vi "getAllsubset.vi"(8 "error in (no error)":errorcluster, 10 "getAll":T1, 11 "instrument.OptiCool in":refnum<class "instrument.OptiCool.lvclass">) -> (0 "error out":errorcluster, 2 "output cluster":variant, 3 "instrument.OptiCool out":refnum<class "instrument.OptiCool.lvclass">)   [LabVIEW 2019, in "instrument.OptiCool.lvclass"]
uses:
  instrument.OptiCool.lvclass
  instrument.PPMS/Typedefs/PPMS.getAll--cluster.ctl
  instrument.PPMS/instrument.PPMS.lvclass
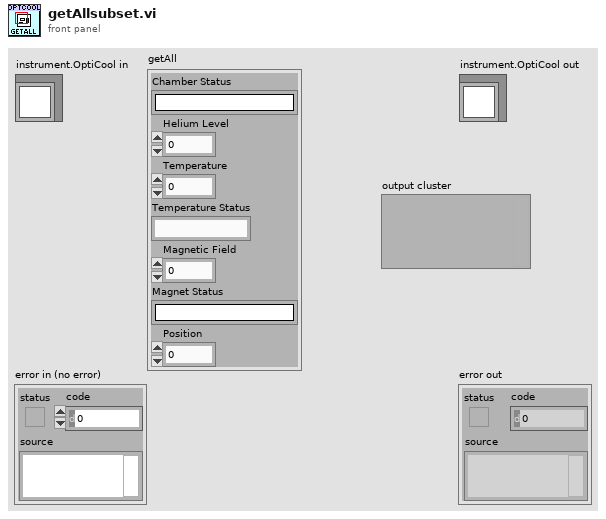
[diagram p1: front panel]
types:
  T1 = typedef "instrument.PPMS.lvclass/PPMS.getAll--cluster.ctl" = cluster{"Chamber Status":string, "Helium Level":dbl, "Temperature":dbl, "Temperature Status":string, "Magnetic Field":dbl, "Magnet Status":string, "Position":dbl}
  T2 = cluster{"Chamber Status":string, "Temperature":dbl, "Temperature Status":string, "Magnetic Field":dbl, "Magnet Status":string}
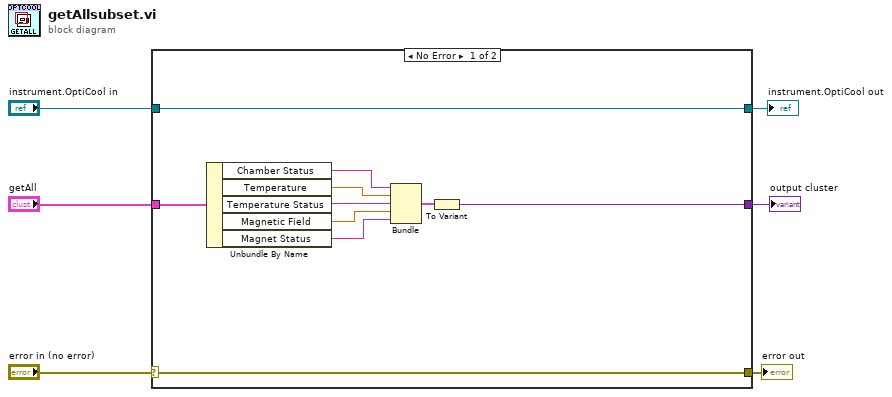
[diagram p0: block diagram]
diagram:
  n1 = case shown="No Error" "error in (no error)" {
    selector: "error in (no error)" -> [w15 w18]
    tunnel: [w15 w18] -> w1
    tunnel: [w16 w17] -> w2
    tunnel: "instrument.OptiCool in" -> [w16 w17]
    tunnel: "getAll" -> [w8 _]
    tunnel: [w14 _] -> w3
    frame No Error {
      n2 = Unbundle By Name(w8) -> ("Chamber Status"=w11:string, "Temperature"=w12:dbl, "Temperature Status"=w13:string, "Magnetic Field"=w10:dbl, "Magnet Status"=w9:string)
      n3 = Bundle("Chamber Status"=w11, "Temperature"=w12, "Temperature Status"=w13, "Magnetic Field"=w10, "Magnet Status"=w9) -> (w7:T2)  [unwired: 1 in]
      n4 = To Variant(anything=w7) -> (Variant=w14:variant)
    }
    frame Error {
    }
  }
  "error out" <- w1
  "instrument.OptiCool out" <- w2
  "output cluster" <- w3
